vi "Get Current Measurement Option.vi"(0 "Capture Load Current Waveform":string, 11 "error in (no error)":errorcluster) -> (4 "Current Measurement Option":T1, 15 "error out":errorcluster)   [LabVIEW 2020, in "LDO Load Transient.lvlib"]
uses:
  LDO Load Transient.lvlib
  Typedefs/Current Measurement Type.ctl
  8909a21a-1569-4915-98bc-16adc36bdd43.vi
  <userlib>/_Soliton/Measurement Suite/Reusables/InstrumentSessionAPIs/SessionManagerApiPath.vi
  <vilib>/Utility/sysdir.llb/Get System Directory.vi
  <vilib>/Utility/LVLibp/Get Exported File Path.vi
  <userlib>/_Soliton/Measurement Suite/Reusables/Errors/Error 6001.vi
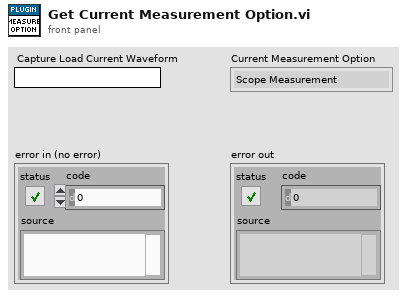
[diagram p1: front panel]
types:
  T1 = typedef "LDO Load Transient.lvlib/Current Measurement Type.ctl" = enum16{"Scope Measurement", "SMU Measurement"}
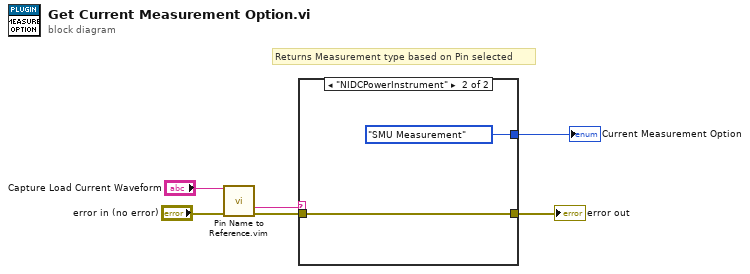
[diagram p0: block diagram]
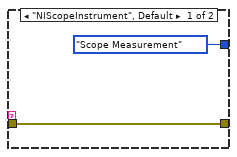
[diagram p2: hidden frame]
diagram:
  # "Returns Measurement type based on Pin selected"
  n1 = call "Pin Name to Reference.vim"("Pin Name"="Capture Load Current Waveform", "error in (no error)"="error in (no error)") -> ("Instr_Type"=w5:string, "error out"=w3:errorcluster)  [unwired: 8 in, 4 out]
  n2 = case shown="\"NIDCPowerInstrument\"" w5 {
    tunnel: w3 -> [w8 w10]
    tunnel: [w8 w10] -> w4
    tunnel: [Current_Measurement_Type."Scope Measurement" Current_Measurement_Type."SMU Measurement"] -> w6
    frame "NIScopeInstrument", Default {
    }
    frame "NIDCPowerInstrument" {
    }
  }
  "Current Measurement Option" <- w6
  "error out" <- w4
